vi "IntakeSubsystem.vi"   [LabVIEW 2017]
uses:
  IntakeCommand.ctl
  RunMode.ctl
  IntakeOutput.ctl
  <vilib>/Rock Robotics/WPI/ThirdParty/Phoenix-LabVIEW/Motor Controller/Controls/CTRE_Phoenix_MotorControl_ControlMode.ctl
panel:
  # "This is responsable for intake control"
types:
  T1 = typedef "IntakeOutput.ctl" = cluster{"Control Mode":T2, "LeftIntakeSetting":dbl, "RightIntakeSetting":dbl}
  T2 = typedef "CTRE_Phoenix_MotorControl_ControlMode.ctl" = u16
  T3 = typedef "IntakeCommand.ctl" = cluster{"Collect":bool, "Deposit":bool, "Mode":T4}
  T4 = typedef "RunMode.ctl" = enum16{"Auto", "Teleop", "Disabled"}
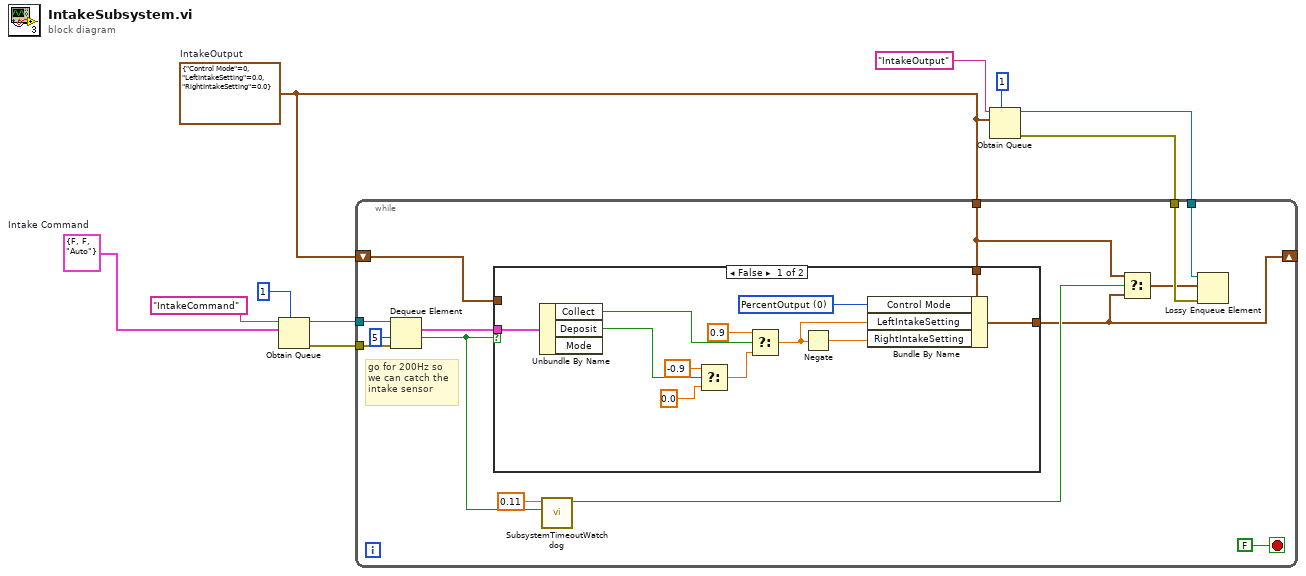
[diagram p0: block diagram]
diagram:
  w3 = T1 {"Control Mode"=0, "LeftIntakeSetting"=0.0, "RightIntakeSetting"=0.0}  # IntakeOutput
  w6 = T3 {"Collect"=FALSE, "Deposit"=FALSE, "Mode"=enum."Auto"}  # Intake Command
  n1 = Obtain Queue(max queue size (-1, unlimited)=1, name (unnamed)="IntakeCommand", element data type=w6) -> (queue out=w8:refnum<queue>, error out=w7:errorcluster)  [unwired: 2 in, 1 out]
  n2 = Obtain Queue(max queue size (-1, unlimited)=1, name (unnamed)="IntakeOutput", element data type=w3) -> (queue out=w2:refnum<queue>, error out=w1:errorcluster)  [unwired: 2 in, 1 out]
  n3 = while {
    tunnel: w8 -> [w23]
    tunnel: w7 -> [w24]
    shift-right: [w12] -> _
    shift-left: w3 -> [w17]
    tunnel: w3 -> [w11]
    tunnel: w2 -> [w16]
    tunnel: w1 -> [w15]
    stop <- FALSE stop-if-true
    # "go for 200Hz so\nwe can catch the\nintake sensor"
    n4 = Dequeue Element(queue=w23, timeout in ms (-1)=5, error in (no error)=w24) -> (element=w18:T3, timed out?=w19:bool)  [unwired: 2 out]
    n5 = case shown="False" w19 {
      tunnel: w18 -> [w36 _]
      tunnel: w17 -> [_ w37]
      tunnel: [w29 w37] -> w12
      tunnel: w11 -> [w28 _]
      frame False {
        w27 = T2 0 items=["PercentOutput"=0, "Position"=1, "Velocity"=2, "Current"=3, "Follower"=5, "MotionProfile"=6, "MotionMagic"=7, "MotionMagicArc"=8, "MotionProfileArc"=10, "Disabled"=15] ("Control Mode")
        n6 = Unbundle By Name(w36) -> ("Collect"=w31:bool, "Deposit"=w30:bool)  [unwired: 1 out]
        n7 = Select(t=-0.9, s=w30, f=0.0) -> (s? t:f=w35:dbl)
        n8 = Select(t=0.9, s=w31, f=w35) -> (s? t:f=w26:dbl)
        n9 = Negate(x=w26) -> (-x=w25:dbl)
        n10 = Bundle By Name(cluster=w28, "Control Mode"=w27, "LeftIntakeSetting"=w26, "RightIntakeSetting"=w25) -> (w29:T1)
      }
      frame True {
      }
    }
    n11 = call "SubsystemTimeoutWatchdog.vi"("Keep counting?"=w19, "Max Timeout (s)"=0.11 ("Time Target (s)")) -> ("Over Max Timeout?"=w13:bool)  [unwired: 9 in]
    n12 = Select(t=w11, s=w13, f=w12) -> (s? t:f=w14:T1)
    n13 = Lossy Enqueue Element(queue=w16, element=w14, error in (no error)=w15) -> ()  [unwired: 4 out]
  }
